vi "EXCEL READ AND WRITE1.vi"(4 "FUNCTION":enum16{"", "READ", "WRITE"}(ring), 5 "POST ACTION":enum16{"", "KEEP OPEN", "CLOSE"}(ring), 6 "RANGE 1":string, 7 "Excel._Application":refnum<k7>, 8 "SHEET NUMBER":dbl, 9 "STR TO WRITE":string, 10 "Path in":path=path "D:/LABVIEW TRIALS/USER.xlsx", 11 "Automation Refnum in":refnum<k7>) -> (2 "STR READ":string, 3 "Path out":path=path "D:/LABVIEW TRIALS/USER.xlsx")   [LabVIEW 2021]
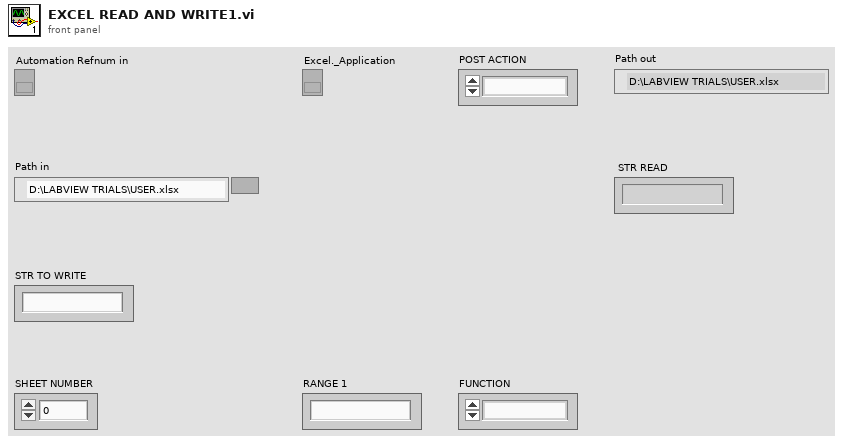
[diagram p1: front panel]
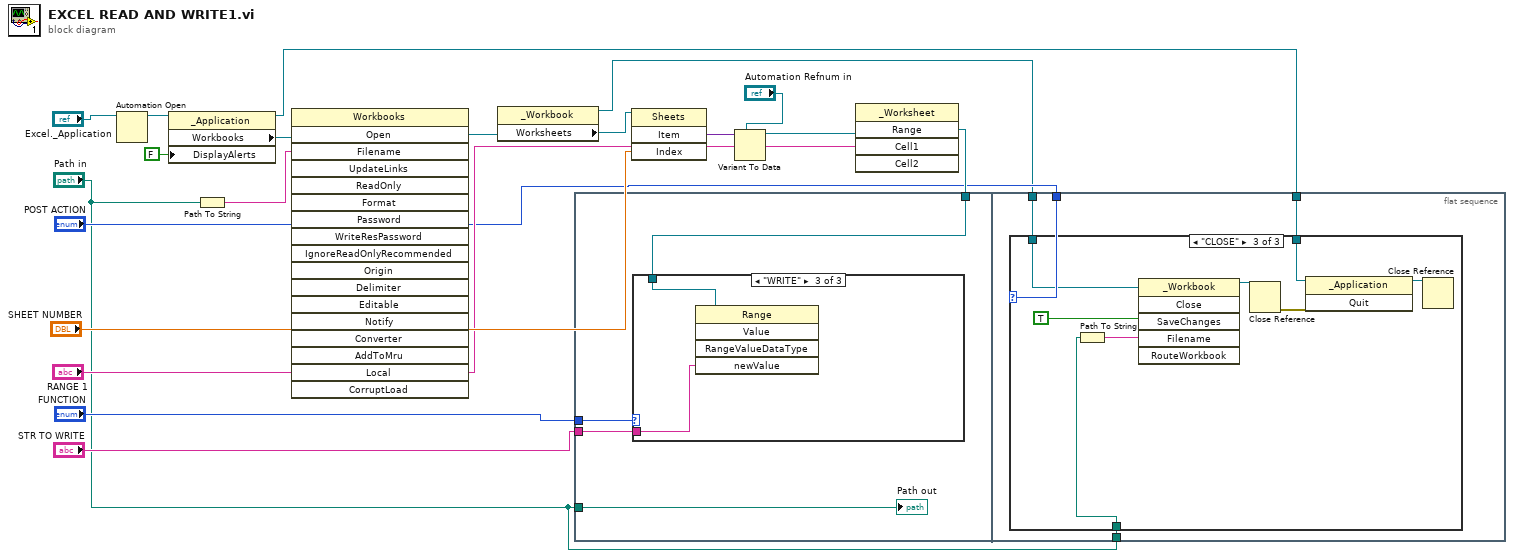
[diagram p0: block diagram]
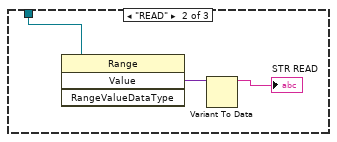
[diagram p3: hidden frame]
diagram:
  n1 = Automation Open(Automation Refnum="Excel._Application") -> (Automation Refnum=w16:refnum<k7>)  [unwired: 3 in, 1 out]
  n2 = property class="_Application"(reference=w16, "DisplayAlerts"=FALSE) -> (reference out=w2:refnum<k7>, "Workbooks"=w15:refnum<k7>)  [unwired: 1 in, 1 out]
  n3 = Path To String(path="Path in") -> (string=w14:string)
  n4 = invoke class="Workbooks" method="Open"(reference=w15, "Filename"=w14) -> ("Open"=w7:refnum<k7>)  [unwired: 16 in, 17 out]
  n5 = property class="_Workbook"(reference=w7) -> (reference out=w3:refnum<k7>, "Worksheets"=w13:refnum<k7>)  [unwired: 1 in, 1 out]
  n6 = flat-sequence {
    tunnel: "FUNCTION" -> [w23]
    tunnel: "STR TO WRITE" -> [w22]
    tunnel: w18 -> [w21]
    tunnel: "Path in" -> [w20]
    tunnel: "POST ACTION" -> [w32]
    tunnel: w3 -> [w31]
    tunnel: w2 -> [w30]
    tunnel: "Path in" -> [w29]
    frame #0 {
      n7 = case shown="\"WRITE\"" w23 {
        tunnel: w21 -> [_ w26 w28]
        tunnel: w22 -> [_ _ w27]
        frame "" {
        }
        frame "READ" {
          n8 = invoke class="Range" method="Value"(reference=w26) -> ("Value"=w25:variant)  [unwired: 3 in, 3 out]
          n9 = Variant To Data(Variant=w25) -> (data=→"STR READ":string)  [unwired: 2 in, 1 out]
        }
        frame "WRITE" {
          n10 = invoke class="Range" method="Value"(reference=w28, "newValue"=w27) -> ()  [unwired: 3 in, 5 out]
        }
      }
      "Path out" <- w20
    }
    frame #1 {
      n11 = case shown="\"CLOSE\"" w32 {
        tunnel: w31 -> [_ _ w40]
        tunnel: w30 -> [_ _ w36]
        tunnel: w29 -> [_ _ w33]
        frame "" {
        }
        frame "KEEP OPEN" {
        }
        frame "CLOSE" {
          n12 = Path To String(path=w33) -> (string=w34:string)
          n13 = invoke class="_Workbook" method="Close"(reference=w40, "SaveChanges"=TRUE, "Filename"=w34) -> (reference out=w38:refnum<k7>)  [unwired: 3 in, 5 out]
          n14 = Close Reference(reference=w38) -> (error out=w37:errorcluster)  [unwired: 1 in]
          n15 = invoke class="_Application" method="Quit"(reference=w36, error in=w37) -> (reference out=w35:refnum<k7>)  [unwired: 1 in, 2 out]
          n16 = Close Reference(reference=w35) -> ()  [unwired: 1 in, 1 out]
        }
      }
    }
  }
  n17 = invoke class="Sheets" method="Item"(reference=w13, "Index"="SHEET NUMBER") -> ("Item"=w11:variant)  [unwired: 2 in, 3 out]
  n18 = Variant To Data(type="Automation Refnum in", Variant=w11) -> (data=w9:refnum<k7>)  [unwired: 1 in, 1 out]
  n19 = invoke class="_Worksheet" method="Range"(reference=w9, "Cell1"="RANGE 1") -> ("Range"=w18:refnum<k7>)  [unwired: 3 in, 4 out]
